vi "F to C.vi"(11 "F":dbl) -> (0 "C":dbl)   [LabVIEW 2021]
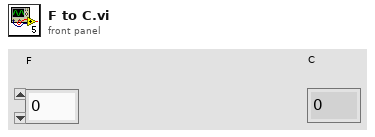
[diagram p1: front panel]
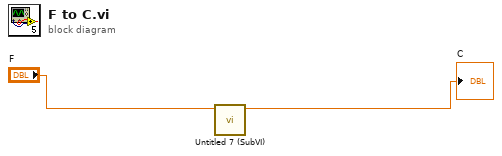
[diagram p0: block diagram]
diagram:
  n1 = call "Untitled 7 (SubVI).vi"("F"="F") -> ("Numeric"=→"C":dbl)  [unwired: 10 in]
